vi "proyecto.vi"() -> ()   [LabVIEW 2017]
uses:
  <vilib>/Instr/_visa.llb/VISA Configure Serial Port (Instr).vi
panel:
  out "?":string
  out "?":string
  out "Medidor de cajas":string
  out "Luxómetro":dbl(knob) scale=0.0..2200.0
  out "Termómetro":dbl(slide) scale=0.0..45.0
  in  "VISA resource name":refnum<visa-resource-name>
  out "PPM:":string
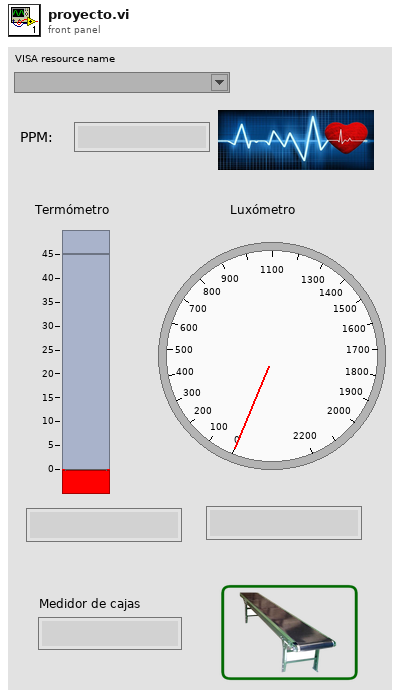
[diagram p1: front panel]
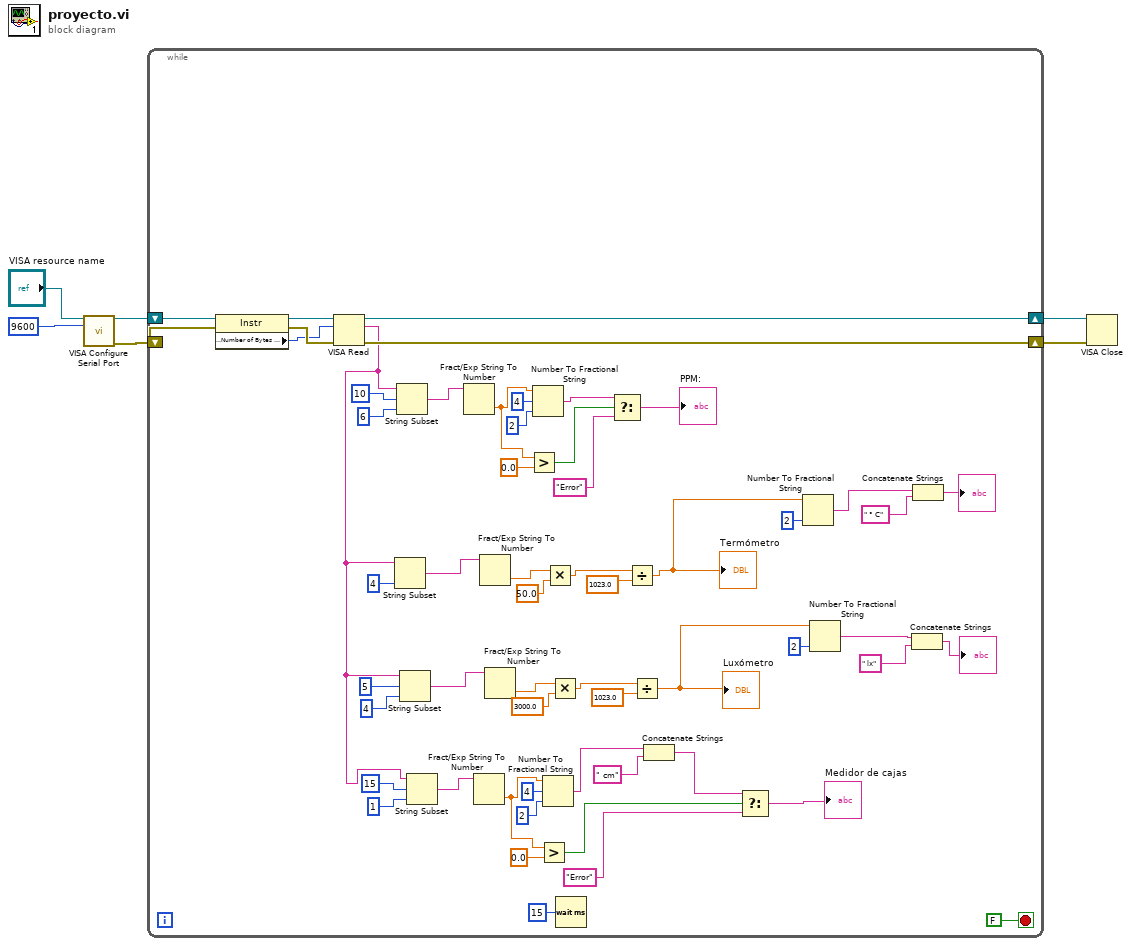
[diagram p0: block diagram]
diagram:
  n1 = call-poly "VISA Configure Serial Port"("VISA resource name"="VISA resource name", "baud rate (9600)"=u32 9600) -> ("VISA resource name out"=w4:refnum<visa-resource-name>, "error out"=w3:errorcluster)  [unwired: 12 in]
  n2 = while {
    shift-right: [w58] -> w2
    shift-left: w4 -> [w63]
    shift-right: [w57] -> w1
    shift-left: w3 -> [w62]
    stop <- FALSE stop-if-true
    n3 = property class="Instr"(reference=w63, error in=w62) -> (reference out=w61:refnum<visa-resource-name>, error out=w60:errorcluster, "Serial Settings:Number of Bytes at Serial Port"=w59:u32)
    n4 = VISA Read(VISA resource name=w61, byte count=w59, error in (no error)=w60) -> (VISA resource name out=w58:refnum<visa-resource-name>, read buffer=w21:string, error out=w57:errorcluster)  [unwired: 1 out]
    n5 = String Subset(string=w21, length (rest)=4 ("length (rest)")) -> (substring=w42:string)  [unwired: 1 in]
    n6 = String Subset(string=w21, offset (0)=10, length (rest)=6 ("length (rest)")) -> (substring=w52:string)
    n7 = String Subset(string=w21, offset (0)=5, length (rest)=4 ("length (rest)")) -> (substring=w33:string)
    n8 = String Subset(string=w21, offset (0)=15, length (rest)=1 ("length (rest)")) -> (substring=w24:string)
    n9 = Fract/Exp String To Number(string=w52) -> (number=w48:dbl)  [unwired: 3 in, 1 out]
    n10 = Fract/Exp String To Number(string=w24) -> (number=w28:dbl)  [unwired: 3 in, 1 out]
    n11 = Fract/Exp String To Number(string=w42) -> (number=w40:dbl)  [unwired: 3 in, 1 out]
    n12 = Fract/Exp String To Number(string=w33) -> (number=w35:dbl)  [unwired: 3 in, 1 out]
    n13 = Greater?(x=w48, y=0.0) -> (0:w47:bool)
    n14 = Number To Fractional String(number=w48, width (-)=i16 4, precision (6)=i16 2) -> (F-format string=w46:string)  [unwired: 1 in]
    n15 = Greater?(x=w28, y=0.0) -> (0:w29:bool)
    n16 = Number To Fractional String(number=w28, width (-)=i16 4, precision (6)=i16 2) -> (F-format string=w18:string)  [unwired: 1 in]
    n17 = Multiply(x=w40, y=50.0) -> (x*y=w38:dbl)
    n18 = Multiply(x=w35, y=3000.0) -> (x*y=w37:dbl)
    n19 = Wait (ms)(milliseconds to wait=u32 15) -> ()  [unwired: 1 out]
    n20 = Select(t=w46, s=w47, f="Error") -> (s? t:f=→"PPM:":string)
    n21 = Divide(x=w38, y=1023.0) -> (x/y=w16:dbl)
    "Termómetro" <- w16
    n22 = Divide(x=w37, y=1023.0) -> (x/y=w15:dbl)
    "Luxómetro" <- w15
    n23 = Concatenate Strings(w18, " cm") -> (w19:string)
    n24 = Select(t=w19, s=w29, f="Error") -> (s? t:f=→"Medidor de cajas":string)
    n25 = Number To Fractional String(number=w16, precision (6)=i16 2) -> (F-format string=w8:string)  [unwired: 2 in]
    n26 = Number To Fractional String(number=w15, precision (6)=i16 2) -> (F-format string=w7:string)  [unwired: 2 in]
    n27 = Concatenate Strings(w7, " lx") -> (→"?":string)
    n28 = Concatenate Strings(w8, " ° C") -> (→"?":string)
  }
  n29 = VISA Close(VISA resource name=w2, error in (no error)=w1) -> ()  [unwired: 1 out]
